vi "Kolo.vi"() -> ()   [LabVIEW 2012]
panel:
  out "XY Graph":cluster{"X":dbl, "Y":dbl}[](graph)
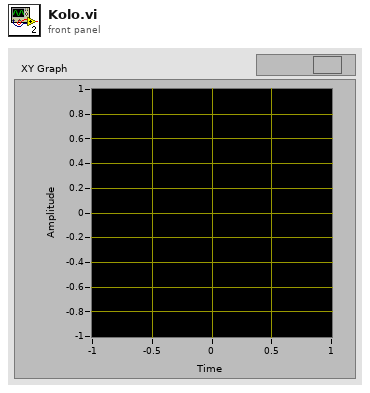
[diagram p1: front panel]
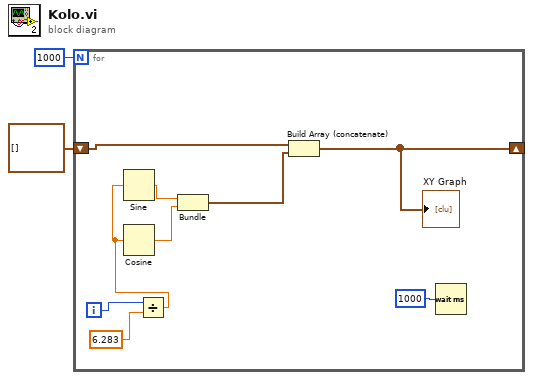
[diagram p0: block diagram]
diagram:
  n1 = for {
    N: 1000 -> [_]
    shift-right: [w3] -> _
    shift-left: cluster{dbl, dbl}[] [] -> [w10]
    i -> [w8]
    n2 = Divide(x=w8, y=6.283) -> (x/y=w5:dbl)
    n3 = Sine(x=w5) -> (sin(x)=w7:dbl)
    n4 = Cosine(x=w5) -> (cos(x)=w6:dbl)
    n5 = Bundle(w7, w6) -> (w11:cluster{dbl, dbl})  [unwired: 1 in]
    n6 = Build Array (concatenate)(w10, w11) -> (w3:cluster{dbl, dbl}[])
    "XY Graph" <- w3
    n7 = Wait (ms)(milliseconds to wait=u32 1000) -> ()  [unwired: 1 out]
  }
